vi "Set_Measurement_Conditions.vi"(3 "Simulate/Run":T3, 4 "Currently on Point":i32=11, 5 "Traverse line":T5 {"Carrier_2 Q (l/min)" format="%#.2f"; "Row Duration (mins)" format="%#.1f"; "Row No" min=0; "Trace Gas Concentration (%)" min=0.0 format="%#_4f"; "Carrier_1 Q (l/min)" format="%#.2f"; "Tunnel Speed" format="%#.2f"; "Start X" format="%#.2f"; "Start Y" format="%#.2f"; "Start Z" format="%#.2f"; "End X" format="%#.2f"; "End Y" format="%#.2f"; "End Z" format="%#.2f"; "Averaging time (min)" min=0.0 format="%#.2f"}) -> (0 "Status Cluster":T1)   [LabVIEW 2014]
uses:
  Traverse_cluster.ctl
  Spacing.ctl
  Controls/Multi_run_mode.ctl
  Execute_case.ctl
  Controls/User_Specific_mode.ctl
  Status_Cluster.ctl
  Multi_Run_Status.ctl
  ADAM Client/Sub VIs/ADAM Controls/Client_Source_Status.ctl
  Globals/Preference_global.vi
  Globals/Extra_Commands_Global.vi
panel:
  out "Heaters On?":bool
  out "Time Source Started":dbl
  out "Execute Case":T4=enum."Set All Conditions"
  # "X           Y            Z"
  # "Start"
  # "End"
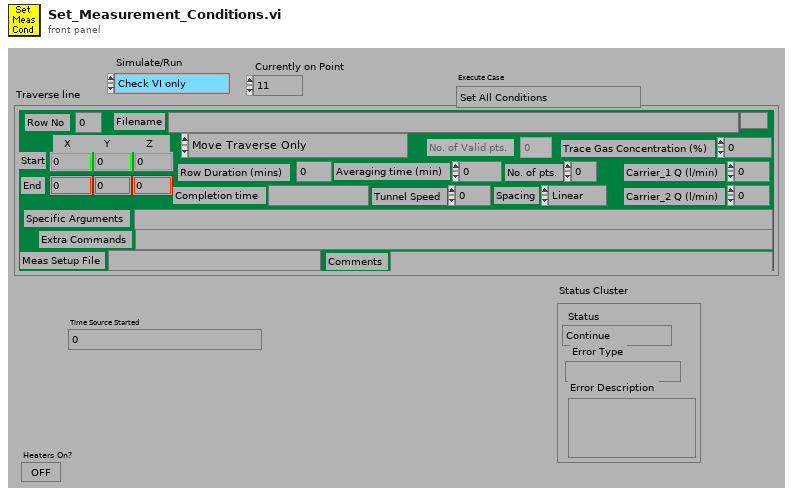
[diagram p1: front panel]
types:
  T1 = typedef "Status_Cluster.ctl" = cluster{"Status":T2, "Error Type":string, "Error Description":string}
  T2 = typedef "Multi_Run_Status.ctl" = enum16{"Continue", "Jump to Next Point", "Jump to Next Row", "Jump To Fall Back", "Terminate Run"}
  T3 = typedef "User_Specific_mode.ctl" = enum16{"Check VI only", "Run VI"}
  T4 = typedef "Execute_case.ctl" = enum16{"Start", "EnFlo Tunnel Check", "Set All Conditions", "Establish Exp Conditions", "The End"}
  T5 = typedef "Traverse_cluster.ctl" = cluster{"Start X":sgl, "Start Y":sgl, "Start Z":sgl, "End X":sgl, "End Y":sgl, "End Z":sgl, "No. of pts.":i32, "Spacing":T6, "Filename":path, "Tunnel Speed":dbl, "Averaging time (min)":dbl, "Extra Commands":string, "Carrier_1 Q (l/min)":dbl, "Carrier_2 Q (l/min)":dbl, "Trace Gas Concentration (%)":dbl, "Specific Arguments":string, "Comments":string, "Row No":i32, "Row Type Selector":T7, "Completion time":string, "Row Duration (mins)":dbl, "No. of Valid pts.":i32, "Meas Setup File":string}
  T6 = typedef "Spacing.ctl" = enum16{"Linear", "Log", "Gauss", "Specified", "N/A"}
  T7 = typedef "Multi_run_mode.ctl" = enum16{"Move Traverse Only", "Set Tunnel Speed Only", "Set Source Only", "Set Measurement Conditions", "Single Measurement", "Vertical Profile", "Lateral Profile", "Longitudinal Profile", "Explore Volume", "Multi-Axis Profile", "Auto Calibrate", "Meas Fast FID Bkgnd", "Check Beam Power", "Scanning Valve Measurement", "Run VI Named:", "Set ADAM Ch", "Wait (minutes)", "Send Message", "Synchronize With:", "Fall Back to this Row", "Turn Off Row Repeating", "Blank Row", "Traverse 3D Volume"}
  T8 = typedef "Client_Source_Status.ctl" = enum16{"Not Using", "Using", "Must Have"}
  T9 = typedef "Server_Comms.ctl" = enum16{"Server Link Healthy", "Do Not Link To Server"}
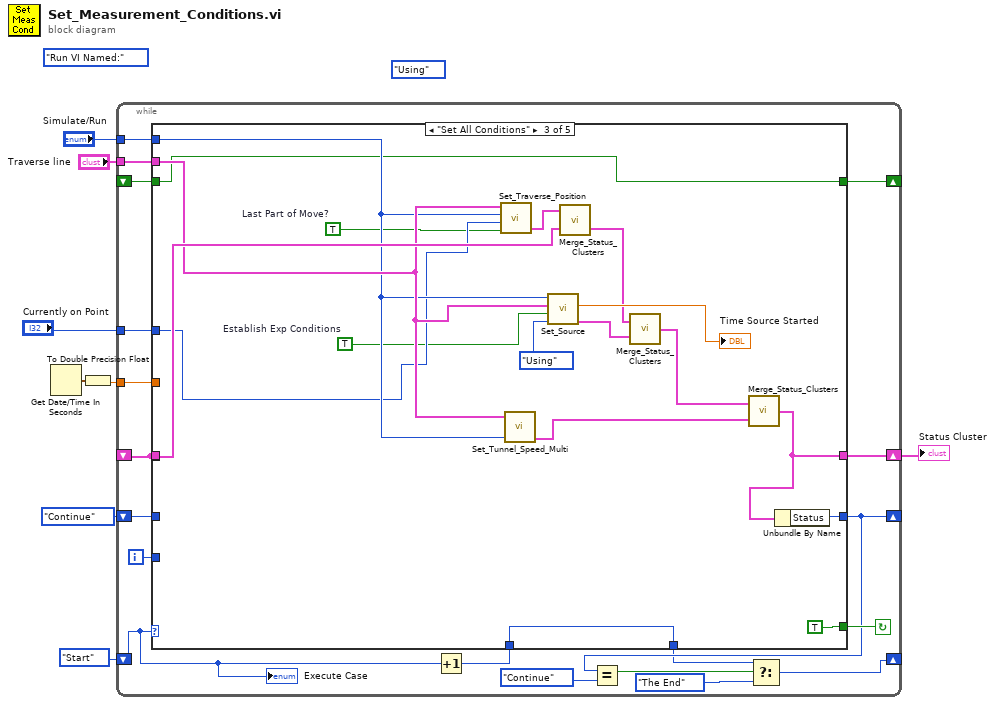
[diagram p0: block diagram]
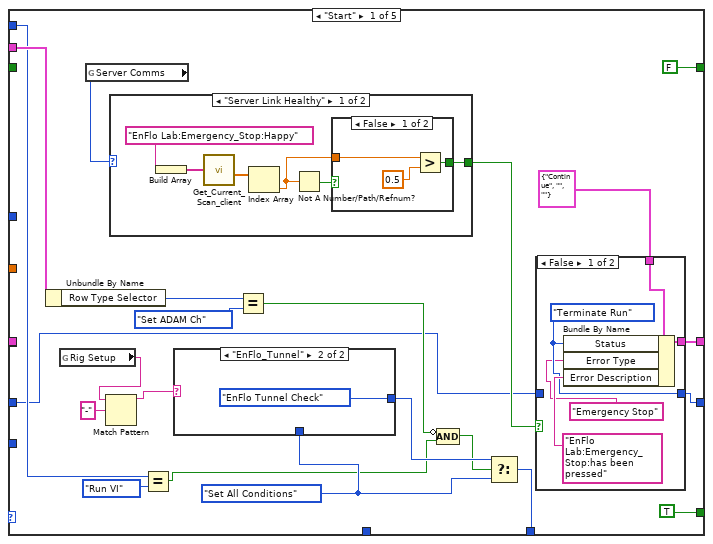
[diagram p2: hidden frame]
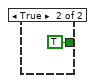
[diagram p4: hidden frame]
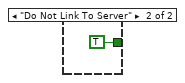
[diagram p5: hidden frame]
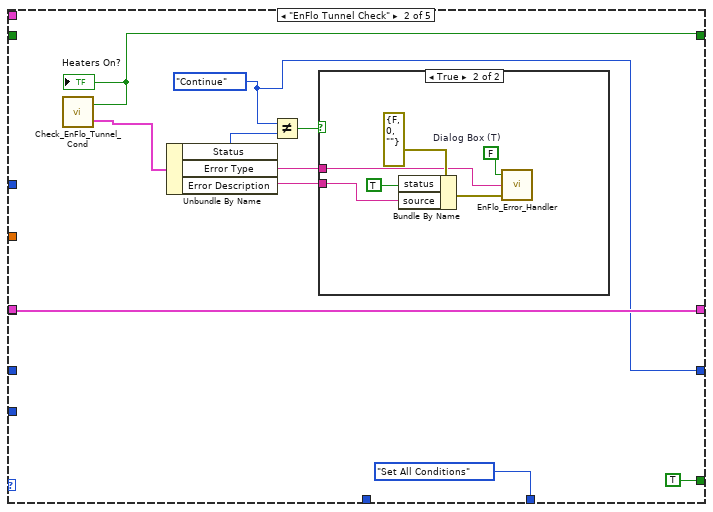
[diagram p7: hidden frame]
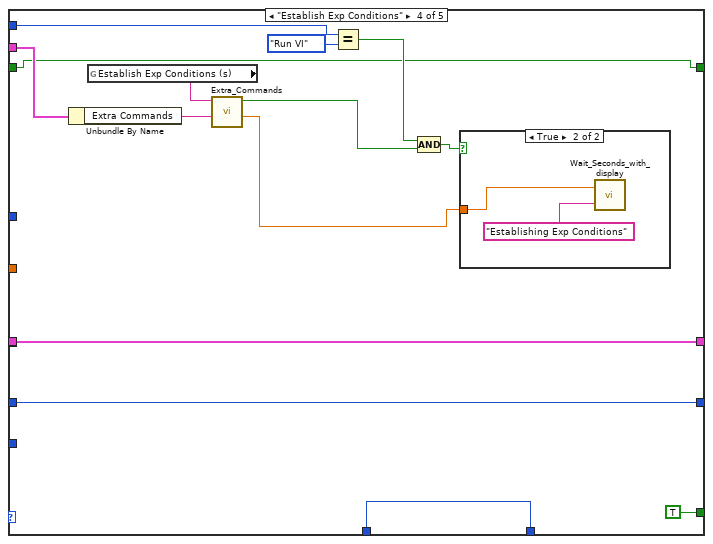
[diagram p9: hidden frame]
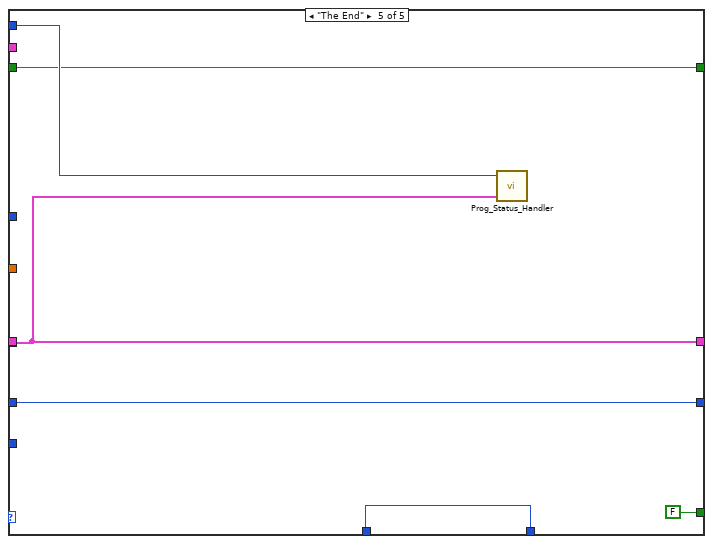
[diagram p11: hidden frame]
diagram:
  (unwired) Client_Source_Status."Using" ("Source Status")
  (unwired) Multi_run_mode."Run VI Named:" ("Mode")
  n1 = Get Date/Time In Seconds() -> (seconds since 1Jan1904=w1:timestamp)
  n2 = To Double Precision Float(number=w1) -> (double precision float=w2:dbl)
  n3 = while {
    tunnel: w2 -> [w12]
    tunnel: "Traverse line" -> [w13]
    tunnel: "Currently on Point" -> [w14]
    shift-left: _ -> [w15]
    shift-right: [w22] -> w4
    shift-left: Multi_Run_Status."Continue" ("Status") -> [w23]
    shift-right: [w21] -> _
    tunnel: "Simulate/Run" -> [w24]
    shift-left: Execute_case."Start" ("Execute Case") -> [w25]
    shift-right: [w17] -> _
    shift-right: [w10] -> _
    shift-left: _ -> [w9]
    i -> [w11]
    stop <- w27 continue-if-true
    n4 = Increment(x=w25) -> (x+1=w26:T4)
    n5 = case shown="\"Set All Conditions\"" w25 {
      tunnel: [TRUE TRUE TRUE TRUE FALSE] -> w27
      tunnel: w26 -> [_ _ w98 w108 w124]
      tunnel: w24 -> [w47 _ w95 w116 w122]
      tunnel: w23 -> [w28 _ _ w107 w123]
      tunnel: w15 -> [_ w74 w102 w106 w120]
      tunnel: [w31 w74 w99 w106 w120] -> w22
      tunnel: [w29 w71 w96 w107 w123] -> w21
      tunnel: [w44 Execute_case."Set All Conditions" ("Execute Case") w98 w108 w124] -> w16
      tunnel: w15 -> [_ _ _ _ _]
      tunnel: w14 -> [_ _ w94 _ _]
      tunnel: w13 -> [w49 _ w101 w115 _]
      tunnel: w12 -> [_ _ _ _ _]
      tunnel: w11 -> [_ _ _ _ _]
      tunnel: [FALSE w70 w91 w105 w121] -> w10
      tunnel: w9 -> [_ _ w91 w105 w121]
      frame "Start" {
        w45 = Execute_case."Set All Conditions" ("Execute Case")
        n6 = Unbundle By Name(w49) -> ("Row Type Selector"=w39:T7)
        n7 = global read "Preference_global.vi" "Rig Setup"() -> (w37:string)
        n8 = global read "Preference_global.vi" "Server Comms"() -> (w34:T9)
        n9 = Match Pattern(string=w37, regular expression="-") -> (before substring=w36:string)  [unwired: 4 out]
        n10 = case shown="\"Server Link Healthy\"" w34 {
          tunnel: [w57 TRUE] -> w33
          frame "Server Link Healthy" {
            n11 = Build Array("EnFlo Lab:Emergency_Stop:Happy") -> (w60:string[])
            n12 = call "Get_Current_Scan_client.vi"("ADAM Ch Names"=w60) -> ("Numerical Values"=w62:dbl[])  [unwired: 1 in, 2 out]
            n13 = Index Array(array=w62) -> (element=w58:dbl)  [unwired: 1 in]
            n14 = Not A Number/Path/Refnum?(number/path/refnum=w58) -> (NaN/Path/Refnum?=w59:bool)
            n15 = case shown="False" w59 {
              tunnel: w58 -> [w65 _]
              tunnel: [w63 TRUE] -> w57
              frame False {
                n16 = Greater?(x=w65, y=0.5) -> (0:w63:bool)
              }
              frame True {
              }
            }
          }
          frame "Do Not Link To Server" {
          }
        }
        n17 = Equal?(x=w47, y=User_Specific_mode."Run VI" ("Simulate/Run")) -> (x = y?=w41:bool)
        n18 = case shown="\"EnFlo_Tunnel\"" w36 {
          tunnel: [w68 Execute_case."EnFlo Tunnel Check" ("Execute Case")] -> w46
          tunnel: w45 -> [w68 _]
          frame "Other", Default {
          }
          frame "EnFlo_Tunnel" {
          }
        }
        n19 = Equal?(x=w39, y=Multi_run_mode."Set ADAM Ch" ("Mode")) -> (x = y?=w42:bool)
        n20 = Compound Arithmetic op=AND(invert w42, w41) -> (w40:bool)
        n21 = Select(t=w46, s=w40, f=w45) -> (s? t:f=w44:T4)
        n22 = case shown="False" w33 {
          tunnel: T1 {"Status"=enum."Continue", "Error Type"="", "Error Description"=""} ("Status Cluster") -> [w54 w55]
          tunnel: [w53 w55] -> w31
          tunnel: [w51 w56] -> w29
          tunnel: w28 -> [_ w56]
          frame False {
            w51 = Multi_Run_Status."Terminate Run" ("Status")
            n23 = Bundle By Name(cluster=w54, "Status"=w51, "Error Type"="Emergency Stop", "Error Description"="EnFlo Lab:Emergency_Stop:has been pressed") -> (w53:T1)
          }
          frame True {
          }
        }
      }
      frame "EnFlo Tunnel Check" {
        w71 = Multi_Run_Status."Continue" ("Status")
        n24 = call "Check_EnFlo_Tunnel_Cond.vi"() -> ("Status Cluster"=w77:T1, "Heaters On?"=w70:bool)  [unwired: 2 in]
        "Heaters On?" <- w70
        n25 = Unbundle By Name(w77) -> ("Status"=w73:T2, "Error Type"=w76:string, "Error Description"=w75:string)
        n26 = Not Equal?(x=w71, y=w73) -> (x != y?=w72:bool)
        n27 = case shown="True" w72 {
          tunnel: w76 -> [_ w81]
          tunnel: w75 -> [_ w80]
          frame False {
          }
          frame True {
            w83 = FALSE  # Dialog Box (T)
            n28 = Bundle By Name(cluster=errorcluster {"status"=FALSE, "code"=0, "source"=""} ("error in (no error)"), "status"=TRUE ("Bundle Element"), "source"=w80) -> (w84:errorcluster)
            n29 = call "EnFlo_Error_Handler.vi"("error in (no error)"=w84, "Error Type"=w81, "Dialog Box (T)"=w83) -> ()  [unwired: 3 out]
          }
        }
      }
      frame "Set All Conditions" {
        w86 = TRUE  # Last Part of Move?
        w87 = TRUE  # Establish Exp Conditions
        n30 = call "Set_Traverse_Position.vi"("Last Part of Move?"=w86, "Currently on Point"=w94, "Simulate/Run"=w95, "Traverse line"=w101) -> ("Status Cluster"=w88:T1)  [unwired: 2 in]
        n31 = call "Set_Tunnel_Speed_Multi.vi"("Simulate/Run"=w95, "Traverse line"=w101) -> ("Status Cluster"=w100:T1)  [unwired: 3 out]
        n32 = call "Set_Source.vi"("Source Status"=Client_Source_Status."Using", "Establish Exp Conditions"=w87, "Traverse line"=w101, "Simulate/Run"=w95) -> ("Status Cluster"=w89:T1, "Time Source Started"=→"Time Source Started":dbl)  [unwired: 4 out]
        n33 = call "Merge_Status_Clusters.vi"("Status Cluster 2"=w102, "Status Cluster 1"=w88) -> ("Status Cluster Out"=w93:T1)
        n34 = call "Merge_Status_Clusters.vi"("Status Cluster 2"=w89, "Status Cluster 1"=w93) -> ("Status Cluster Out"=w92:T1)
        n35 = call "Merge_Status_Clusters.vi"("Status Cluster 2"=w100, "Status Cluster 1"=w92) -> ("Status Cluster Out"=w99:T1)
        n36 = Unbundle By Name(w99) -> ("Status"=w96:T2)
      }
      frame "Establish Exp Conditions" {
        n37 = Unbundle By Name(w115) -> ("Extra Commands"=w109:string)
        n38 = global read "Extra_Commands_Global.vi" "Establish Exp Conditions (s)"() -> (w114:string)
        n39 = call "Extra_Commands.vi"("String to Search"=w109, "Command"=w114) -> ("Numeric Value"=w104:dbl, "Command Found"=w111:bool)  [unwired: 1 in, 3 out]
        n40 = Equal?(x=w116, y=User_Specific_mode."Run VI" ("Simulate/Run")) -> (x = y?=w110:bool)
        n41 = Compound Arithmetic op=AND(w110, w111) -> (w112:bool)
        n42 = case shown="True" w112 {
          tunnel: w104 -> [_ w118]
          frame False {
          }
          frame True {
            n43 = call "Wait_Seconds_with_display.vi"("Message"="Establishing Exp Conditions", "Seconds to wait"=w118) -> ()  [unwired: 2 out]
          }
        }
      }
      frame "The End" {
        n44 = call "Prog_Status_Handler.vi"("Status Cluster"=w120, "Simulate/Run"=w122) -> ()  [unwired: 2 out]
      }
    }
    n45 = Equal?(x=w21, y=Multi_Run_Status."Continue" ("Status")) -> (x = y?=w19:bool)
    n46 = Select(t=w16, s=w19, f=Execute_case."The End" ("Execute Case")) -> (s? t:f=w17:T4)
    "Execute Case" <- w25
  }
  "Status Cluster" <- w4
